vi "compute_zernike_coeffs_starter.vi"() -> ()   [LabVIEW 2020]
uses:
  HasoSlopes.lvclass
  Pupil.lvclass
  ModalCoef.lvclass
panel:
  out "Zernike pupil":i32[][](graph)
  out "Zernike Coefficients":sgl[](graph)
  in  "Haso slopes file name":string="Data\\data_phase_computation.has"
  out "error out":errorcluster
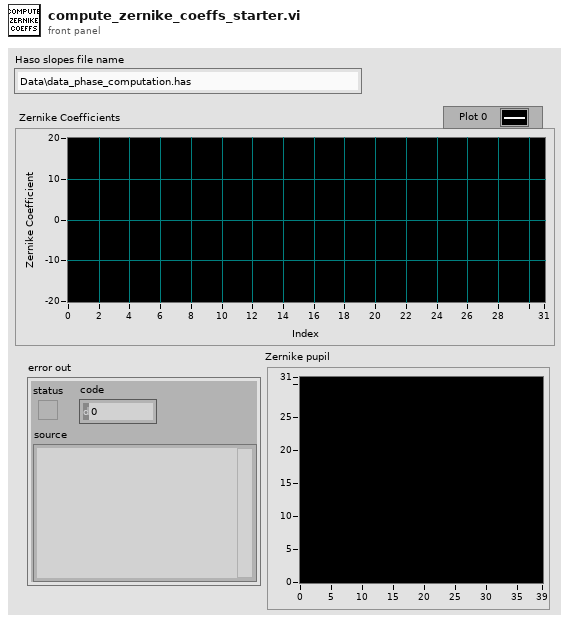
[diagram p1: front panel]
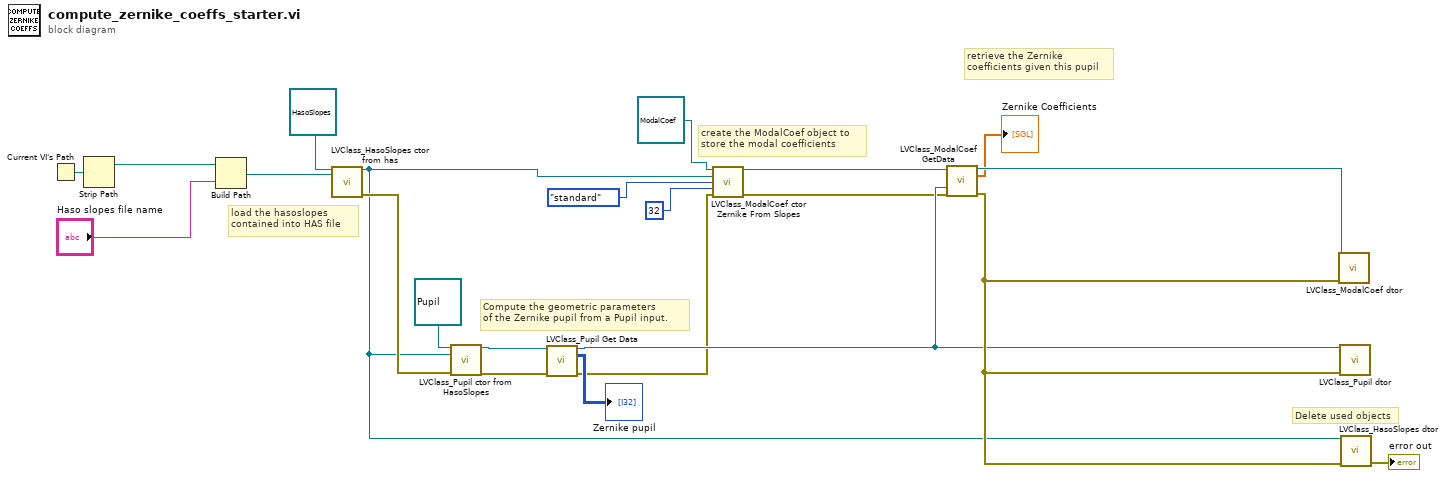
[diagram p0: block diagram]
diagram:
  # "Delete used objects"
  # "retrieve the Zernike\ncoefficients given this pupil"
  # "create the ModalCoef object to\nstore the modal coefficients"
  # "Compute the geometric parameters\nof the Zernike pupil from a Pupil input."
  # "load the hasoslopes\ncontained into HAS file"
  n1 = Current VI's Path() -> (path=w17:path)
  n2 = Strip Path(path=w17) -> (stripped path=w14:path)  [unwired: 1 out]
  n3 = Build Path(base path=w14, name or relative path="Haso slopes file name") -> (appended path=w15:path)
  n4 = call "LVClass_HasoSlopes ctor from has.vi"("HasoSlopes (const)"=refnum<class "HasoSlopes.lvclass"> refnum ("HasoSlopes in"), ".has path"=w15) -> ("HasoSlopes (new)"=w3:refnum<class "HasoSlopes.lvclass">, "error out"=w13:errorcluster)  [unwired: 12 in]
  n5 = call "LVClass_Pupil ctor from HasoSlopes.vi"("Pupil (const)"=refnum<class "Pupil.lvclass"> refnum ("Pupil in"), "HasoSlopes"=w3, "error in (no error)"=w13) -> ("Pupil (new)"=w8:refnum<class "Pupil.lvclass">, "error out"=w7:errorcluster)  [unwired: 10 in, 1 out]
  n6 = call "LVClass_Pupil Get Data.vi"("Pupil in"=w8, "error in (no error)"=w7) -> ("Pupil out"=w10:refnum<class "Pupil.lvclass">, "Data"=→"Zernike pupil":i32[][], "error out"=w6:errorcluster)  [unwired: 11 in]
  n7 = call "LVClass_ModalCoef ctor Zernike From Slopes.vi"("ModalCoef (const)"=refnum<class "ModalCoef.lvclass"> refnum ("ModalCoef in"), "HasoSlopes"=w3, "normalization"=enum16{"standard", "rms"}."standard", "nb_coefs"=u32 32, "error in (no error)"=w6) -> ("ModalCoef (new)"=w5:refnum<class "ModalCoef.lvclass">, "error out"=w4:errorcluster)  [unwired: 9 in]
  n8 = call "LVClass_ModalCoef GetData.vi"("ModalCoef in"=w5, "Pupil.lvclass"=w10, "error in (no error)"=w4) -> ("ModalCoef out"=w19:refnum<class "ModalCoef.lvclass">, "coef"=→"Zernike Coefficients":sgl[], "error out"=w20:errorcluster)  [unwired: 8 in, 2 out]
  n9 = call "LVClass_ModalCoef dtor.vi"("ModalCoef in"=w19, "error in (no error)"=w20) -> ()  [unwired: 12 in, 2 out]
  n10 = call "LVClass_Pupil dtor.vi"("Pupil in"=w10, "error in (no error)"=w20) -> ()  [unwired: 12 in, 2 out]
  n11 = call "LVClass_HasoSlopes dtor.vi"("HasoSlopes in"=w3, "error in (no error)"=w20) -> ("error out"=→"error out":errorcluster)  [unwired: 12 in, 1 out]
